vi "VTI read msg.vi"(8 "error in (no error)":errorcluster, 10 "Initialized?":bool, 11 "Queue in":T2) -> (0 "error out":errorcluster, 1 "timed out?":bool, 2 "Data":variant, 3 "Command":T1)   [LabVIEW 2024, in "Temperature controller.lvlib"]
uses:
  Temperature controller.lvlib
  Messenger service/Data types/Modul ref.ctl
  ctl/TC commands.ctl
  ctl/MSG for VTI.ctl
  Messenger service/MessengerLib.lvlib
panel:
  out "x-y":u32
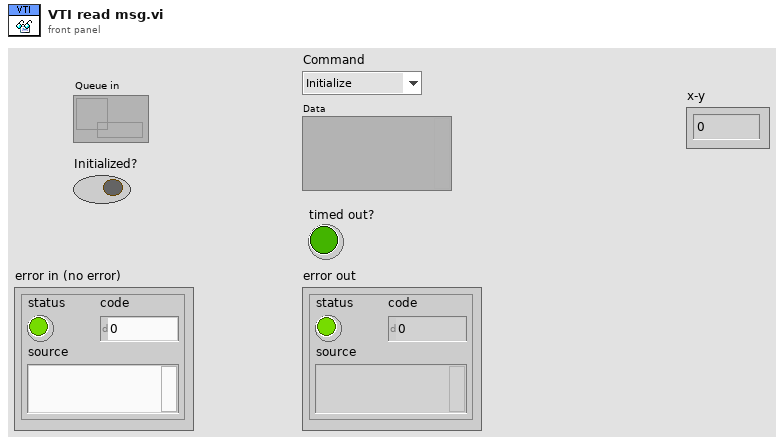
[diagram p1: front panel]
types:
  T1 = typedef "Temperature controller.lvlib/TC commands.ctl" = enum16{"Initialize", "Update", "Stop tmp change", "Set temperature", "Set point", "Disconnect", "End", "Ignore"}
  T2 = typedef "MessengerLib.lvlib/Modul ref.ctl" = refnum<queue>
  T3 = typedef "Temperature controller.lvlib/MSG for VTI.ctl" = cluster{"Command":T1, "Data":variant}
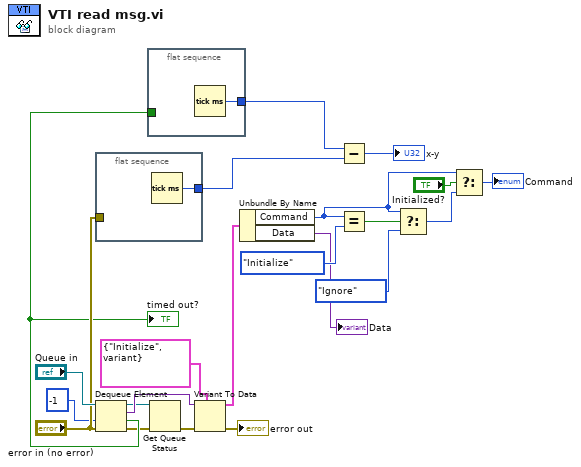
[diagram p0: block diagram]
diagram:
  n1 = flat-sequence {
    tunnel: [w23] -> w8
    tunnel: "error in (no error)" -> [_]
    frame #0 {
      n2 = Tick Count (ms)() -> (millisecond timer value=w23:u32)
    }
  }
  n3 = Dequeue Element(queue="Queue in", timeout in ms (-1)=-1, error in (no error)="error in (no error)") -> (queue out=w1:T2, element=w19:variant, timed out?=w4:bool, error out=w2:errorcluster)
  "timed out?" <- w4
  n4 = flat-sequence {
    tunnel: [w24] -> w9
    tunnel: w4 -> [_]
    frame #0 {
      n5 = Tick Count (ms)() -> (millisecond timer value=w24:u32)
    }
  }
  n6 = Get Queue Status(queue=w1, error in (no error)=w2) -> (error out=w18:errorcluster)  [unwired: 1 in, 7 out]
  n7 = Variant To Data(error in=w18, type=T3 {"Command"=enum."Initialize", "Data"=variant}, Variant=w19) -> (data=w21:T3, error out=→"error out":errorcluster)
  n8 = Unbundle By Name(w21) -> ("Command"=w14:T1, "Data"=→"Data":variant)
  n9 = Subtract(x=w9, y=w8) -> (x-y=→"x-y":u32)
  n10 = Equal?(x=w14, y=TC_commands."Initialize" ("x")) -> (x = y?=w15:bool)
  n11 = Select(t=w14, s=w15, f=TC_commands."Ignore") -> (s? t:f=w12:T1)
  n12 = Select(t=w14, s="Initialized?", f=w12) -> (s? t:f=→"Command":T1)
